vi "Robocopy.vi"(4 "Output summary to LabVIEW (will no longer be able to see progress in CMD prompt)":bool, 5 "Folder list":string[](array[string])=["2018", "2017", "2016", "2015", "2014", "2013", "2012", "2011", "2010", "2009", "2008", "2007", "2006", "2005", "2004", "2003", "2002", "2001", "2000", "1999", "1998", "1997", "Preferences"], 6 "Dest. drive root":path=path "G:/", 7 "Source drive root":path=path "Z:/", 8 "Mode of operation":u16(ring) items=["One way mirror, overwrite destination files even if newer", "One way mirror, don't overwrite newer files at destination", "Two way copy, newest files at both locations"]) -> (0 "Errors out":errorcluster[](array[cluster]), 1 "Commands":string[](array[string]), 3 "End summary":string[](array[string]))   [LabVIEW 2017]
panel:
  # "PN 10/12/2014, \n       16/12/2015"
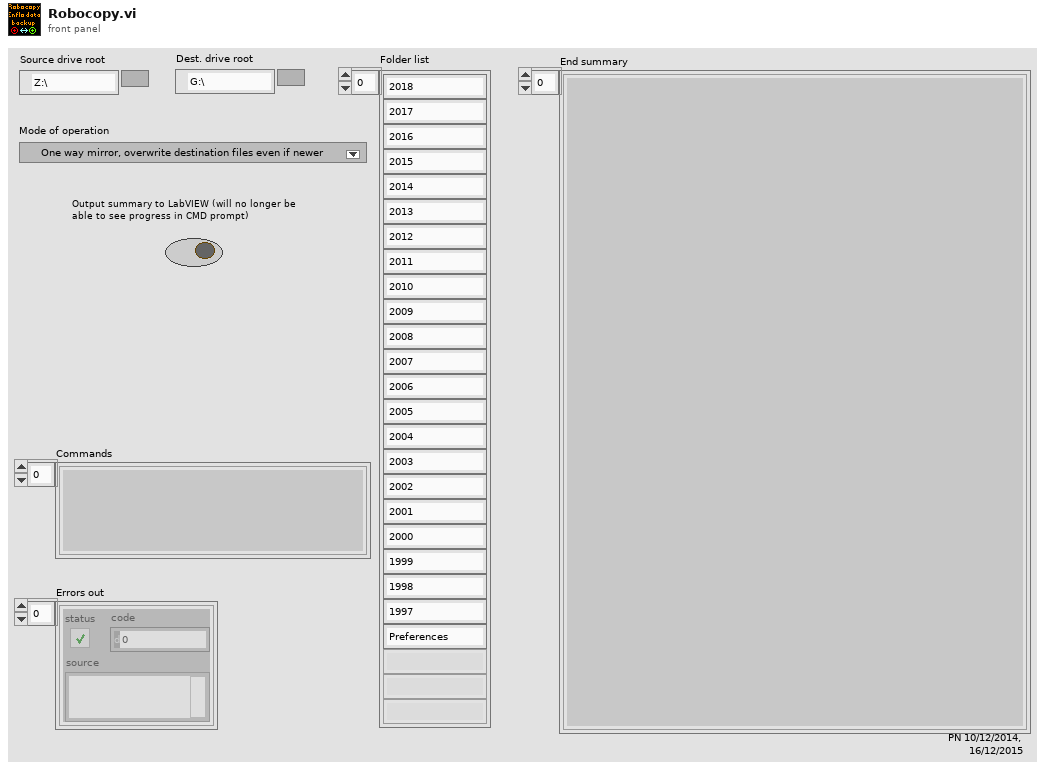
[diagram p1: front panel]
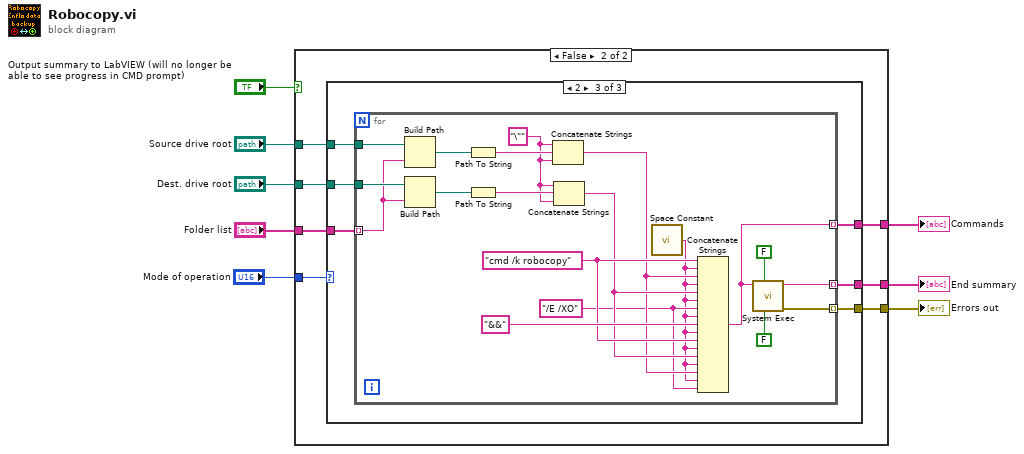
[diagram p0: block diagram]
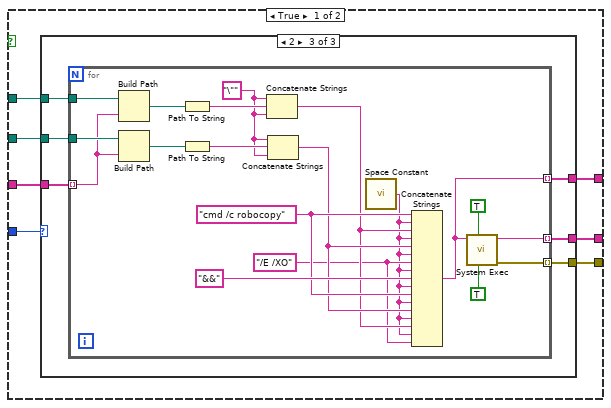
[diagram p2: hidden frame]
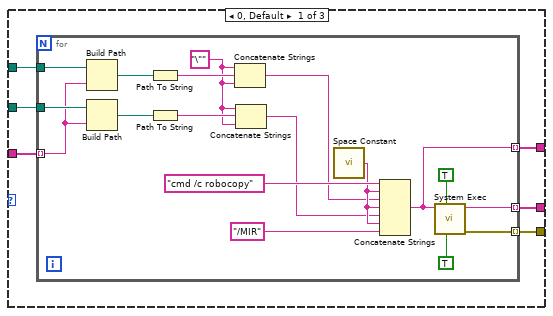
[diagram p3: hidden frame]
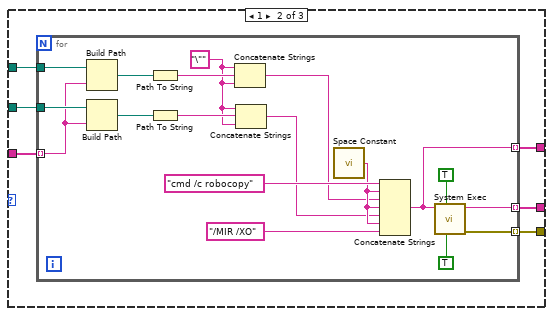
[diagram p4: hidden frame]
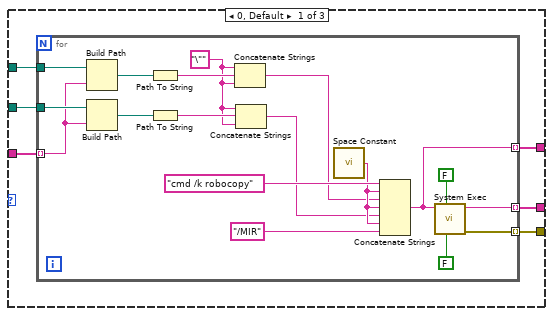
[diagram p5: hidden frame]
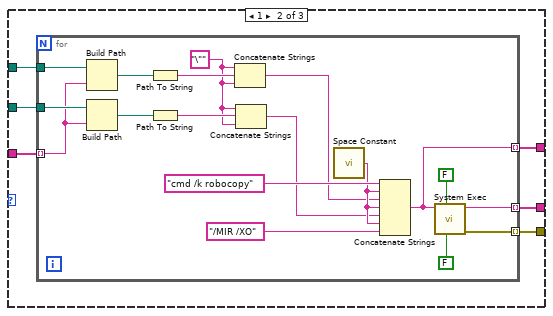
[diagram p6: hidden frame]
diagram:
  n1 = case shown="False" "Output summary to LabVIEW (will no longer be able to see progress in CMD prompt)" {
    tunnel: "Source drive root" -> [w15 w95]
    tunnel: "Dest. drive root" -> [w14 w94]
    tunnel: "Folder list" -> [w13 w93]
    tunnel: "Mode of operation" -> [w12 w92]
    tunnel: [w11 w91] -> w4
    tunnel: [w10 w90] -> w3
    tunnel: [w9 w89] -> w2
    frame True {
      n2 = case shown="2" w12 {
        tunnel: w15 -> [w21 w45 w69]
        tunnel: w14 -> [w20 w44 w68]
        tunnel: w13 -> [w19 w43 w67]
        tunnel: [w18 w42 w66] -> w10
        tunnel: [w17 w41 w64] -> w11
        tunnel: [w16 w40 w65] -> w9
        frame 0, Default {
          n3 = for {
            tunnel: w21 -> [w37]
            tunnel: w20 -> [w36]
            tunnel: w19 -> [w35] mode=indexing
            tunnel: [w30] -> w17 mode=indexing
            tunnel: [w23] -> w18 mode=indexing
            tunnel: [w22] -> w16 mode=indexing
            w24 = "\"" ("string")
            n4 = Build Path(base path=w37, name or relative path=w35) -> (appended path=w33:path)
            n5 = Build Path(base path=w36, name or relative path=w35) -> (appended path=w32:path)
            n6 = Path To String(path=w33) -> (string=w28:string)
            n7 = Path To String(path=w32) -> (string=w26:string)
            n8 = Concatenate Strings(w24, w28, w24) -> (w27:string)
            n9 = Concatenate Strings(w24, w26, w24) -> (w25:string)
            n10 = call <vilib>:"Space Constant.vi"() -> ("String"=w29:string)
            n11 = Concatenate Strings("cmd /c robocopy", w29, w27, w29, w25, w29, "/MIR" ("string")) -> (w23:string)
            n12 = call <vilib>:"System Exec.vi"("run minimized? (F)"=TRUE, "wait until completion? (T)"=TRUE, "command line"=w23) -> ("error out"=w30:errorcluster, "standard output"=w22:string)  [unwired: 5 in, 2 out]
          }
        }
        frame 1 {
          n13 = for {
            tunnel: w45 -> [w61]
            tunnel: w44 -> [w60]
            tunnel: w43 -> [w59] mode=indexing
            tunnel: [w54] -> w41 mode=indexing
            tunnel: [w47] -> w42 mode=indexing
            tunnel: [w46] -> w40 mode=indexing
            w48 = "\"" ("string")
            n14 = Build Path(base path=w61, name or relative path=w59) -> (appended path=w57:path)
            n15 = Build Path(base path=w60, name or relative path=w59) -> (appended path=w56:path)
            n16 = Path To String(path=w57) -> (string=w52:string)
            n17 = Path To String(path=w56) -> (string=w50:string)
            n18 = Concatenate Strings(w48, w52, w48) -> (w51:string)
            n19 = Concatenate Strings(w48, w50, w48) -> (w49:string)
            n20 = call <vilib>:"Space Constant.vi"() -> ("String"=w53:string)
            n21 = Concatenate Strings("cmd /c robocopy", w53, w51, w53, w49, w53, "/MIR /XO" ("string")) -> (w47:string)
            n22 = call <vilib>:"System Exec.vi"("run minimized? (F)"=TRUE, "wait until completion? (T)"=TRUE, "command line"=w47) -> ("error out"=w54:errorcluster, "standard output"=w46:string)  [unwired: 5 in, 2 out]
          }
        }
        frame 2 {
          n23 = for {
            tunnel: w69 -> [w86]
            tunnel: w68 -> [w85]
            tunnel: w67 -> [w84] mode=indexing
            tunnel: [w78] -> w66 mode=indexing
            tunnel: [w77] -> w65 mode=indexing
            tunnel: [w71] -> w64 mode=indexing
            w79 = "\"" ("string")
            w72 = "/E /XO" ("string")
            w75 = "cmd /c robocopy"
            n24 = Build Path(base path=w86, name or relative path=w84) -> (appended path=w83:path)
            n25 = Build Path(base path=w85, name or relative path=w84) -> (appended path=w82:path)
            n26 = Path To String(path=w83) -> (string=w81:string)
            n27 = Path To String(path=w82) -> (string=w80:string)
            n28 = Concatenate Strings(w79, w81, w79) -> (w73:string)
            n29 = Concatenate Strings(w79, w80, w79) -> (w74:string)
            n30 = call <vilib>:"Space Constant.vi"() -> ("String"=w70:string)
            n31 = Concatenate Strings(w75, w70, w73, w70, w74, w70, w72, w70, "&&" ("string"), w70, w75, w70, w74, w70, w73, w70, w72) -> (w78:string)
            n32 = call <vilib>:"System Exec.vi"("run minimized? (F)"=TRUE, "wait until completion? (T)"=TRUE, "command line"=w78) -> ("error out"=w71:errorcluster, "standard output"=w77:string)  [unwired: 5 in, 2 out]
          }
        }
      }
    }
    frame False {
      n33 = case shown="2" w92 {
        tunnel: w95 -> [w101 w125 w149]
        tunnel: w94 -> [w100 w124 w148]
        tunnel: w93 -> [w99 w123 w147]
        tunnel: [w98 w122 w146] -> w90
        tunnel: [w97 w121 w144] -> w91
        tunnel: [w96 w120 w145] -> w89
        frame 0, Default {
          n34 = for {
            tunnel: w101 -> [w117]
            tunnel: w100 -> [w116]
            tunnel: w99 -> [w115] mode=indexing
            tunnel: [w110] -> w97 mode=indexing
            tunnel: [w103] -> w98 mode=indexing
            tunnel: [w102] -> w96 mode=indexing
            w104 = "\"" ("string")
            n35 = Build Path(base path=w117, name or relative path=w115) -> (appended path=w113:path)
            n36 = Build Path(base path=w116, name or relative path=w115) -> (appended path=w112:path)
            n37 = Path To String(path=w113) -> (string=w108:string)
            n38 = Path To String(path=w112) -> (string=w106:string)
            n39 = Concatenate Strings(w104, w108, w104) -> (w107:string)
            n40 = Concatenate Strings(w104, w106, w104) -> (w105:string)
            n41 = call <vilib>:"Space Constant.vi"() -> ("String"=w109:string)
            n42 = Concatenate Strings("cmd /k robocopy", w109, w107, w109, w105, w109, "/MIR" ("string")) -> (w103:string)
            n43 = call <vilib>:"System Exec.vi"("run minimized? (F)"=FALSE, "wait until completion? (T)"=FALSE, "command line"=w103) -> ("error out"=w110:errorcluster, "standard output"=w102:string)  [unwired: 5 in, 2 out]
          }
        }
        frame 1 {
          n44 = for {
            tunnel: w125 -> [w141]
            tunnel: w124 -> [w140]
            tunnel: w123 -> [w139] mode=indexing
            tunnel: [w134] -> w121 mode=indexing
            tunnel: [w127] -> w122 mode=indexing
            tunnel: [w126] -> w120 mode=indexing
            w128 = "\"" ("string")
            n45 = Build Path(base path=w141, name or relative path=w139) -> (appended path=w137:path)
            n46 = Build Path(base path=w140, name or relative path=w139) -> (appended path=w136:path)
            n47 = Path To String(path=w137) -> (string=w132:string)
            n48 = Path To String(path=w136) -> (string=w130:string)
            n49 = Concatenate Strings(w128, w132, w128) -> (w131:string)
            n50 = Concatenate Strings(w128, w130, w128) -> (w129:string)
            n51 = call <vilib>:"Space Constant.vi"() -> ("String"=w133:string)
            n52 = Concatenate Strings("cmd /k robocopy", w133, w131, w133, w129, w133, "/MIR /XO" ("string")) -> (w127:string)
            n53 = call <vilib>:"System Exec.vi"("run minimized? (F)"=FALSE, "wait until completion? (T)"=FALSE, "command line"=w127) -> ("error out"=w134:errorcluster, "standard output"=w126:string)  [unwired: 5 in, 2 out]
          }
        }
        frame 2 {
          n54 = for {
            tunnel: w149 -> [w166]
            tunnel: w148 -> [w165]
            tunnel: w147 -> [w164] mode=indexing
            tunnel: [w158] -> w146 mode=indexing
            tunnel: [w157] -> w145 mode=indexing
            tunnel: [w151] -> w144 mode=indexing
            w159 = "\"" ("string")
            w152 = "/E /XO" ("string")
            w155 = "cmd /k robocopy"
            n55 = Build Path(base path=w166, name or relative path=w164) -> (appended path=w163:path)
            n56 = Build Path(base path=w165, name or relative path=w164) -> (appended path=w162:path)
            n57 = Path To String(path=w163) -> (string=w161:string)
            n58 = Path To String(path=w162) -> (string=w160:string)
            n59 = Concatenate Strings(w159, w161, w159) -> (w153:string)
            n60 = Concatenate Strings(w159, w160, w159) -> (w154:string)
            n61 = call <vilib>:"Space Constant.vi"() -> ("String"=w150:string)
            n62 = Concatenate Strings(w155, w150, w153, w150, w154, w150, w152, w150, "&&" ("string"), w150, w155, w150, w154, w150, w153, w150, w152) -> (w158:string)
            n63 = call <vilib>:"System Exec.vi"("run minimized? (F)"=FALSE, "wait until completion? (T)"=FALSE, "command line"=w158) -> ("error out"=w151:errorcluster, "standard output"=w157:string)  [unwired: 5 in, 2 out]
          }
        }
      }
    }
  }
  "Errors out" <- w4
  "Commands" <- w3
  "End summary" <- w2
